vi "WILT.vi"() -> ()   [LabVIEW 2016] (continued)
        n1786 = call "WILT Station Controller.vi"("Station Number"=w3862, "GUI Aisle in"=w3864, "Drying Time (Min)"=w3846, "Current Threshold"=w3852, "Station Test State In"=w3857, "Error In"=w3861, "Aisle Location Index"=w3859, "Cool Down Period (seconds)"=w3847, "Disable Flood Check"=w3842, "Delay After Cutout (sec)"=w3844, "Previous Run Statistics"=w3848, "Send Restart Every? (Sec)"=w3849, "Agilent Valve and Switch Locations"=w3853, "Injection Times"=w3855, "Enable Start Retry"=w3850, "Day/Night Cycle"=w3854, "Final Start Presses"=w3843, "Semaphore"=w3845) -> ("GUI Aisle 1"=w3863:T3[], "Test Station Out"=w3858:T7, "Enable Start Retry Out"=w3851:bool[], "Error Out"=w3860:errorcluster)  [unwired: 5 in, 1 out]
        n1787 = Bundle By Name(cluster=w3866, "GUI Aisle 3."=w3863, "Station Test State Cluster"=w3858, "Enable Start Retry Array"=w3851) -> (w3865:T24)
        n1788 = call <vilib>:"Add State(s) to Queue__jki_lib_state_machine.vi"("State(s) in (\"\")"=w3868) -> ("States Out"=w3867:string)  [unwired: 14 in]
      }
      frame "Station 42" {
        w3886 = 9  # Aisle Location Index
        w3889 = u32 42  # Station Number
        # "Control the state of station 42"
        n1789 = Unbundle By Name(w3893) -> ("Enable Start Retry Array"=w3878:bool[], "Agilent Switches"=w3880:T2[], "GUI Aisle 3."=w3891:T3[], "Drying Time (Min)"=w3873:dbl[], "Current Threshold"=w3879:dbl, "Station Test State Cluster"=w3884:T7, "Station Timeout Values (1-56) Seconds"=w3874:dbl[], "Send Restart Every? (Sec)"=w3876:dbl, "Injection Times Input"=w3882:T15, "Day/Night Cycle Input"=w3881:T11)
        n1790 = local read "Delay After Cutout (Sec)"() -> (w3871:dbl)
        n1791 = local read "Previous Run Statistics"() -> (w3875:T9[])
        n1792 = local read "Agilent Semaphore"() -> (w3872:T1[])
        n1793 = local read "Disable Flood Check"() -> (w3869:bool)
        n1794 = local read "Final Start Presses"() -> (w3870:i32)
        n1795 = call "WILT Station Controller.vi"("Station Number"=w3889, "GUI Aisle in"=w3891, "Drying Time (Min)"=w3873, "Current Threshold"=w3879, "Station Test State In"=w3884, "Error In"=w3888, "Aisle Location Index"=w3886, "Cool Down Period (seconds)"=w3874, "Disable Flood Check"=w3869, "Delay After Cutout (sec)"=w3871, "Previous Run Statistics"=w3875, "Send Restart Every? (Sec)"=w3876, "Agilent Valve and Switch Locations"=w3880, "Injection Times"=w3882, "Enable Start Retry"=w3878, "Day/Night Cycle"=w3881, "Final Start Presses"=w3870, "Semaphore"=w3872) -> ("GUI Aisle 1"=w3890:T3[], "Test Station Out"=w3885:T7, "Enable Start Retry Out"=w3877:bool[], "Error Out"=w3887:errorcluster)  [unwired: 5 in, 1 out]
        n1796 = Bundle By Name(cluster=w3893, "GUI Aisle 3."=w3890, "Station Test State Cluster"=w3885, "Enable Start Retry Array"=w3877) -> (w3892:T24)
        n1797 = call <vilib>:"Add State(s) to Queue__jki_lib_state_machine.vi"("State(s) in (\"\")"=w3895) -> ("States Out"=w3894:string)  [unwired: 14 in]
      }
      frame "Station 43" {
        w3913 = 10  # Aisle Location Index
        w3916 = u32 43  # Station Number
        # "Control the state of station 43"
        n1798 = Unbundle By Name(w3920) -> ("Enable Start Retry Array"=w3905:bool[], "Agilent Switches"=w3907:T2[], "GUI Aisle 3."=w3918:T3[], "Drying Time (Min)"=w3900:dbl[], "Current Threshold"=w3906:dbl, "Station Test State Cluster"=w3911:T7, "Station Timeout Values (1-56) Seconds"=w3901:dbl[], "Send Restart Every? (Sec)"=w3903:dbl, "Injection Times Input"=w3909:T15, "Day/Night Cycle Input"=w3908:T11)
        n1799 = local read "Previous Run Statistics"() -> (w3902:T9[])
        n1800 = local read "Delay After Cutout (Sec)"() -> (w3898:dbl)
        n1801 = local read "Disable Flood Check"() -> (w3896:bool)
        n1802 = local read "Agilent Semaphore"() -> (w3899:T1[])
        n1803 = local read "Final Start Presses"() -> (w3897:i32)
        n1804 = call "WILT Station Controller.vi"("Station Number"=w3916, "GUI Aisle in"=w3918, "Drying Time (Min)"=w3900, "Current Threshold"=w3906, "Station Test State In"=w3911, "Error In"=w3915, "Aisle Location Index"=w3913, "Cool Down Period (seconds)"=w3901, "Disable Flood Check"=w3896, "Delay After Cutout (sec)"=w3898, "Previous Run Statistics"=w3902, "Send Restart Every? (Sec)"=w3903, "Agilent Valve and Switch Locations"=w3907, "Injection Times"=w3909, "Enable Start Retry"=w3905, "Day/Night Cycle"=w3908, "Final Start Presses"=w3897, "Semaphore"=w3899) -> ("GUI Aisle 1"=w3917:T3[], "Test Station Out"=w3912:T7, "Enable Start Retry Out"=w3904:bool[], "Error Out"=w3914:errorcluster)  [unwired: 5 in, 1 out]
        n1805 = call <vilib>:"Add State(s) to Queue__jki_lib_state_machine.vi"("State(s) in (\"\")"=w3922) -> ("States Out"=w3921:string)  [unwired: 14 in]
        n1806 = Bundle By Name(cluster=w3920, "GUI Aisle 3."=w3917, "Station Test State Cluster"=w3912, "Enable Start Retry Array"=w3904) -> (w3919:T24)
      }
      frame "Station 44" {
        w3940 = 11  # Aisle Location Index
        w3943 = u32 44  # Station Number
        # "Control the state of station 44"
        n1807 = Unbundle By Name(w3947) -> ("Enable Start Retry Array"=w3932:bool[], "Agilent Switches"=w3934:T2[], "GUI Aisle 3."=w3945:T3[], "Drying Time (Min)"=w3927:dbl[], "Current Threshold"=w3933:dbl, "Station Test State Cluster"=w3938:T7, "Station Timeout Values (1-56) Seconds"=w3928:dbl[], "Send Restart Every? (Sec)"=w3930:dbl, "Injection Times Input"=w3936:T15, "Day/Night Cycle Input"=w3935:T11)
        n1808 = local read "Previous Run Statistics"() -> (w3929:T9[])
        n1809 = local read "Disable Flood Check"() -> (w3923:bool)
        n1810 = local read "Delay After Cutout (Sec)"() -> (w3925:dbl)
        n1811 = local read "Agilent Semaphore"() -> (w3926:T1[])
        n1812 = local read "Final Start Presses"() -> (w3924:i32)
        n1813 = call "WILT Station Controller.vi"("Station Number"=w3943, "GUI Aisle in"=w3945, "Drying Time (Min)"=w3927, "Current Threshold"=w3933, "Station Test State In"=w3938, "Error In"=w3942, "Aisle Location Index"=w3940, "Cool Down Period (seconds)"=w3928, "Disable Flood Check"=w3923, "Delay After Cutout (sec)"=w3925, "Previous Run Statistics"=w3929, "Send Restart Every? (Sec)"=w3930, "Agilent Valve and Switch Locations"=w3934, "Injection Times"=w3936, "Enable Start Retry"=w3932, "Day/Night Cycle"=w3935, "Final Start Presses"=w3924, "Semaphore"=w3926) -> ("GUI Aisle 1"=w3944:T3[], "Test Station Out"=w3939:T7, "Enable Start Retry Out"=w3931:bool[], "Error Out"=w3941:errorcluster)  [unwired: 5 in, 1 out]
        n1814 = Bundle By Name(cluster=w3947, "GUI Aisle 3."=w3944, "Station Test State Cluster"=w3939, "Enable Start Retry Array"=w3931) -> (w3946:T24)
        n1815 = call <vilib>:"Add State(s) to Queue__jki_lib_state_machine.vi"("State(s) in (\"\")"=w3949) -> ("States Out"=w3948:string)  [unwired: 14 in]
      }
      frame "Station 45" {
        w3967 = 0  # Aisle Location Index
        w3970 = u32 45  # Station Number
        # "Control the state of station 45"
        n1816 = Unbundle By Name(w3974) -> ("Enable Start Retry Array"=w3958:bool[], "Agilent Switches"=w3961:T2[], "GUI Aisle 4."=w3972:T3[], "Drying Time (Min)"=w3954:dbl[], "Current Threshold"=w3960:dbl, "Station Test State Cluster"=w3965:T7, "Station Timeout Values (1-56) Seconds"=w3955:dbl[], "Send Restart Every? (Sec)"=w3957:dbl, "Injection Times Input"=w3963:T15, "Day/Night Cycle Input"=w3962:T11)
        n1817 = local read "Delay After Cutout (Sec)"() -> (w3952:dbl)
        n1818 = local read "Previous Run Statistics"() -> (w3956:T9[])
        n1819 = local read "Agilent Semaphore"() -> (w3953:T1[])
        n1820 = local read "Disable Flood Check"() -> (w3950:bool)
        n1821 = local read "Final Start Presses"() -> (w3951:i32)
        n1822 = call "WILT Station Controller.vi"("Station Number"=w3970, "GUI Aisle in"=w3972, "Drying Time (Min)"=w3954, "Current Threshold"=w3960, "Station Test State In"=w3965, "Error In"=w3969, "Aisle Location Index"=w3967, "Cool Down Period (seconds)"=w3955, "Disable Flood Check"=w3950, "Delay After Cutout (sec)"=w3952, "Previous Run Statistics"=w3956, "Send Restart Every? (Sec)"=w3957, "Agilent Valve and Switch Locations"=w3961, "Injection Times"=w3963, "Enable Start Retry"=w3958, "Day/Night Cycle"=w3962, "Final Start Presses"=w3951, "Semaphore"=w3953) -> ("GUI Aisle 1"=w3971:T3[], "Test Station Out"=w3966:T7, "Enable Start Retry Out"=w3959:bool[], "Error Out"=w3968:errorcluster)  [unwired: 5 in, 1 out]
        n1823 = Bundle By Name(cluster=w3974, "GUI Aisle 4."=w3971, "Station Test State Cluster"=w3966, "Enable Start Retry Array"=w3959) -> (w3973:T24)
        n1824 = call <vilib>:"Add State(s) to Queue__jki_lib_state_machine.vi"("State(s) in (\"\")"=w3976) -> ("States Out"=w3975:string)  [unwired: 14 in]
      }
      frame "Station 46" {
        w3994 = 1  # Aisle Location Index
        w3997 = u32 46  # Station Number
        # "Control the state of station 46"
        n1825 = Unbundle By Name(w4001) -> ("Enable Start Retry Array"=w3985:bool[], "Agilent Switches"=w3988:T2[], "GUI Aisle 4."=w3999:T3[], "Drying Time (Min)"=w3981:dbl[], "Current Threshold"=w3987:dbl, "Station Test State Cluster"=w3992:T7, "Station Timeout Values (1-56) Seconds"=w3982:dbl[], "Send Restart Every? (Sec)"=w3984:dbl, "Injection Times Input"=w3990:T15, "Day/Night Cycle Input"=w3989:T11)
        n1826 = local read "Delay After Cutout (Sec)"() -> (w3979:dbl)
        n1827 = local read "Final Start Presses"() -> (w3978:i32)
        n1828 = local read "Agilent Semaphore"() -> (w3980:T1[])
        n1829 = local read "Previous Run Statistics"() -> (w3983:T9[])
        n1830 = local read "Disable Flood Check"() -> (w3977:bool)
        n1831 = call "WILT Station Controller.vi"("Station Number"=w3997, "GUI Aisle in"=w3999, "Drying Time (Min)"=w3981, "Current Threshold"=w3987, "Station Test State In"=w3992, "Error In"=w3996, "Aisle Location Index"=w3994, "Cool Down Period (seconds)"=w3982, "Disable Flood Check"=w3977, "Delay After Cutout (sec)"=w3979, "Previous Run Statistics"=w3983, "Send Restart Every? (Sec)"=w3984, "Agilent Valve and Switch Locations"=w3988, "Injection Times"=w3990, "Enable Start Retry"=w3985, "Day/Night Cycle"=w3989, "Final Start Presses"=w3978, "Semaphore"=w3980) -> ("GUI Aisle 1"=w3998:T3[], "Test Station Out"=w3993:T7, "Enable Start Retry Out"=w3986:bool[], "Error Out"=w3995:errorcluster)  [unwired: 5 in, 1 out]
        n1832 = Bundle By Name(cluster=w4001, "GUI Aisle 4."=w3998, "Station Test State Cluster"=w3993, "Enable Start Retry Array"=w3986) -> (w4000:T24)
        n1833 = call <vilib>:"Add State(s) to Queue__jki_lib_state_machine.vi"("State(s) in (\"\")"=w4003) -> ("States Out"=w4002:string)  [unwired: 14 in]
      }
      frame "Station 47" {
        w4021 = 2  # Aisle Location Index
        w4024 = u32 47  # Station Number
        # "Control the state of station 47"
        n1834 = Unbundle By Name(w4028) -> ("Enable Start Retry Array"=w4012:bool[], "Agilent Switches"=w4016:T2[], "GUI Aisle 4."=w4026:T3[], "Drying Time (Min)"=w4009:dbl[], "Current Threshold"=w4015:dbl, "Station Test State Cluster"=w4019:T7, "Station Timeout Values (1-56) Seconds"=w4008:dbl[], "Send Restart Every? (Sec)"=w4011:dbl, "Injection Times Input"=w4017:T15, "Day/Night Cycle Input"=w4014:T11)
        n1835 = local read "Delay After Cutout (Sec)"() -> (w4006:dbl)
        n1836 = local read "Final Start Presses"() -> (w4005:i32)
        n1837 = local read "Agilent Semaphore"() -> (w4007:T1[])
        n1838 = local read "Previous Run Statistics"() -> (w4010:T9[])
        n1839 = local read "Disable Flood Check"() -> (w4004:bool)
        n1840 = call "WILT Station Controller.vi"("Station Number"=w4024, "GUI Aisle in"=w4026, "Drying Time (Min)"=w4009, "Current Threshold"=w4015, "Station Test State In"=w4019, "Error In"=w4023, "Aisle Location Index"=w4021, "Cool Down Period (seconds)"=w4008, "Disable Flood Check"=w4004, "Delay After Cutout (sec)"=w4006, "Previous Run Statistics"=w4010, "Send Restart Every? (Sec)"=w4011, "Agilent Valve and Switch Locations"=w4016, "Injection Times"=w4017, "Enable Start Retry"=w4012, "Day/Night Cycle"=w4014, "Final Start Presses"=w4005, "Semaphore"=w4007) -> ("GUI Aisle 1"=w4025:T3[], "Test Station Out"=w4020:T7, "Enable Start Retry Out"=w4013:bool[], "Error Out"=w4022:errorcluster)  [unwired: 5 in, 1 out]
        n1841 = Bundle By Name(cluster=w4028, "GUI Aisle 4."=w4025, "Station Test State Cluster"=w4020, "Enable Start Retry Array"=w4013) -> (w4027:T24)
        n1842 = call <vilib>:"Add State(s) to Queue__jki_lib_state_machine.vi"("State(s) in (\"\")"=w4030) -> ("States Out"=w4029:string)  [unwired: 14 in]
      }
      frame "Station 48" {
        w4048 = 3  # Aisle Location Index
        w4051 = u32 48  # Station Number
        # "Control the state of station 48"
        n1843 = Unbundle By Name(w4055) -> ("Enable Start Retry Array"=w4040:bool[], "Agilent Switches"=w4042:T2[], "GUI Aisle 4."=w4053:T3[], "Drying Time (Min)"=w4035:dbl[], "Current Threshold"=w4041:dbl, "Station Test State Cluster"=w4046:T7, "Station Timeout Values (1-56) Seconds"=w4036:dbl[], "Send Restart Every? (Sec)"=w4038:dbl, "Injection Times Input"=w4044:T15, "Day/Night Cycle Input"=w4043:T11)
        n1844 = local read "Previous Run Statistics"() -> (w4037:T9[])
        n1845 = local read "Disable Flood Check"() -> (w4031:bool)
        n1846 = local read "Delay After Cutout (Sec)"() -> (w4033:dbl)
        n1847 = local read "Agilent Semaphore"() -> (w4034:T1[])
        n1848 = local read "Final Start Presses"() -> (w4032:i32)
        n1849 = call "WILT Station Controller.vi"("Station Number"=w4051, "GUI Aisle in"=w4053, "Drying Time (Min)"=w4035, "Current Threshold"=w4041, "Station Test State In"=w4046, "Error In"=w4050, "Aisle Location Index"=w4048, "Cool Down Period (seconds)"=w4036, "Disable Flood Check"=w4031, "Delay After Cutout (sec)"=w4033, "Previous Run Statistics"=w4037, "Send Restart Every? (Sec)"=w4038, "Agilent Valve and Switch Locations"=w4042, "Injection Times"=w4044, "Enable Start Retry"=w4040, "Day/Night Cycle"=w4043, "Final Start Presses"=w4032, "Semaphore"=w4034) -> ("GUI Aisle 1"=w4052:T3[], "Test Station Out"=w4047:T7, "Enable Start Retry Out"=w4039:bool[], "Error Out"=w4049:errorcluster)  [unwired: 5 in, 1 out]
        n1850 = Bundle By Name(cluster=w4055, "GUI Aisle 4."=w4052, "Station Test State Cluster"=w4047, "Enable Start Retry Array"=w4039) -> (w4054:T24)
        n1851 = call <vilib>:"Add State(s) to Queue__jki_lib_state_machine.vi"("State(s) in (\"\")"=w4057) -> ("States Out"=w4056:string)  [unwired: 14 in]
      }
      frame "Station 49" {
        w4075 = 4  # Aisle Location Index
        w4078 = u32 49  # Station Number
        # "Control the state of station 49"
        n1852 = Unbundle By Name(w4082) -> ("Enable Start Retry Array"=w4067:bool[], "Agilent Switches"=w4069:T2[], "GUI Aisle 4."=w4080:T3[], "Drying Time (Min)"=w4062:dbl[], "Current Threshold"=w4068:dbl, "Station Test State Cluster"=w4073:T7, "Station Timeout Values (1-56) Seconds"=w4063:dbl[], "Send Restart Every? (Sec)"=w4065:dbl, "Injection Times Input"=w4071:T15, "Day/Night Cycle Input"=w4070:T11)
        n1853 = local read "Previous Run Statistics"() -> (w4064:T9[])
        n1854 = local read "Disable Flood Check"() -> (w4058:bool)
        n1855 = local read "Delay After Cutout (Sec)"() -> (w4060:dbl)
        n1856 = local read "Final Start Presses"() -> (w4059:i32)
        n1857 = local read "Agilent Semaphore"() -> (w4061:T1[])
        n1858 = call "WILT Station Controller.vi"("Station Number"=w4078, "GUI Aisle in"=w4080, "Drying Time (Min)"=w4062, "Current Threshold"=w4068, "Station Test State In"=w4073, "Error In"=w4077, "Aisle Location Index"=w4075, "Cool Down Period (seconds)"=w4063, "Disable Flood Check"=w4058, "Delay After Cutout (sec)"=w4060, "Previous Run Statistics"=w4064, "Send Restart Every? (Sec)"=w4065, "Agilent Valve and Switch Locations"=w4069, "Injection Times"=w4071, "Enable Start Retry"=w4067, "Day/Night Cycle"=w4070, "Final Start Presses"=w4059, "Semaphore"=w4061) -> ("GUI Aisle 1"=w4079:T3[], "Test Station Out"=w4074:T7, "Enable Start Retry Out"=w4066:bool[], "Error Out"=w4076:errorcluster)  [unwired: 5 in, 1 out]
        n1859 = Bundle By Name(cluster=w4082, "GUI Aisle 4."=w4079, "Station Test State Cluster"=w4074, "Enable Start Retry Array"=w4066) -> (w4081:T24)
        n1860 = call <vilib>:"Add State(s) to Queue__jki_lib_state_machine.vi"("State(s) in (\"\")"=w4084) -> ("States Out"=w4083:string)  [unwired: 14 in]
      }
      frame "Station 50" {
        w4102 = 5  # Aisle Location Index
        w4105 = u32 50  # Station Number
        # "Control the state of station 50"
        n1861 = Unbundle By Name(w4109) -> ("Enable Start Retry Array"=w4094:bool[], "Agilent Switches"=w4096:T2[], "GUI Aisle 4."=w4107:T3[], "Drying Time (Min)"=w4089:dbl[], "Current Threshold"=w4095:dbl, "Station Test State Cluster"=w4100:T7, "Station Timeout Values (1-56) Seconds"=w4090:dbl[], "Send Restart Every? (Sec)"=w4092:dbl, "Injection Times Input"=w4098:T15, "Day/Night Cycle Input"=w4097:T11)
        n1862 = local read "Previous Run Statistics"() -> (w4091:T9[])
        n1863 = local read "Disable Flood Check"() -> (w4085:bool)
        n1864 = local read "Delay After Cutout (Sec)"() -> (w4087:dbl)
        n1865 = local read "Final Start Presses"() -> (w4086:i32)
        n1866 = local read "Agilent Semaphore"() -> (w4088:T1[])
        n1867 = call "WILT Station Controller.vi"("Station Number"=w4105, "GUI Aisle in"=w4107, "Drying Time (Min)"=w4089, "Current Threshold"=w4095, "Station Test State In"=w4100, "Error In"=w4104, "Aisle Location Index"=w4102, "Cool Down Period (seconds)"=w4090, "Disable Flood Check"=w4085, "Delay After Cutout (sec)"=w4087, "Previous Run Statistics"=w4091, "Send Restart Every? (Sec)"=w4092, "Agilent Valve and Switch Locations"=w4096, "Injection Times"=w4098, "Enable Start Retry"=w4094, "Day/Night Cycle"=w4097, "Final Start Presses"=w4086, "Semaphore"=w4088) -> ("GUI Aisle 1"=w4106:T3[], "Test Station Out"=w4101:T7, "Enable Start Retry Out"=w4093:bool[], "Error Out"=w4103:errorcluster)  [unwired: 5 in, 1 out]
        n1868 = Bundle By Name(cluster=w4109, "GUI Aisle 4."=w4106, "Station Test State Cluster"=w4101, "Enable Start Retry Array"=w4093) -> (w4108:T24)
        n1869 = call <vilib>:"Add State(s) to Queue__jki_lib_state_machine.vi"("State(s) in (\"\")"=w4111) -> ("States Out"=w4110:string)  [unwired: 14 in]
      }
      frame "Station 51" {
        w4129 = 6  # Aisle Location Index
        w4132 = u32 51  # Station Number
        # "Control the state of station 51"
        n1870 = Unbundle By Name(w4136) -> ("Enable Start Retry Array"=w4121:bool[], "Agilent Switches"=w4123:T2[], "GUI Aisle 4."=w4134:T3[], "Drying Time (Min)"=w4116:dbl[], "Current Threshold"=w4122:dbl, "Station Test State Cluster"=w4127:T7, "Station Timeout Values (1-56) Seconds"=w4117:dbl[], "Send Restart Every? (Sec)"=w4119:dbl, "Injection Times Input"=w4125:T15, "Day/Night Cycle Input"=w4124:T11)
        n1871 = local read "Delay After Cutout (Sec)"() -> (w4114:dbl)
        n1872 = local read "Final Start Presses"() -> (w4113:i32)
        n1873 = local read "Agilent Semaphore"() -> (w4115:T1[])
        n1874 = local read "Previous Run Statistics"() -> (w4118:T9[])
        n1875 = local read "Disable Flood Check"() -> (w4112:bool)
        n1876 = call "WILT Station Controller.vi"("Station Number"=w4132, "GUI Aisle in"=w4134, "Drying Time (Min)"=w4116, "Current Threshold"=w4122, "Station Test State In"=w4127, "Error In"=w4131, "Aisle Location Index"=w4129, "Cool Down Period (seconds)"=w4117, "Disable Flood Check"=w4112, "Delay After Cutout (sec)"=w4114, "Previous Run Statistics"=w4118, "Send Restart Every? (Sec)"=w4119, "Agilent Valve and Switch Locations"=w4123, "Injection Times"=w4125, "Enable Start Retry"=w4121, "Day/Night Cycle"=w4124, "Final Start Presses"=w4113, "Semaphore"=w4115) -> ("GUI Aisle 1"=w4133:T3[], "Test Station Out"=w4128:T7, "Enable Start Retry Out"=w4120:bool[], "Error Out"=w4130:errorcluster)  [unwired: 5 in, 1 out]
        n1877 = Bundle By Name(cluster=w4136, "GUI Aisle 4."=w4133, "Station Test State Cluster"=w4128, "Enable Start Retry Array"=w4120) -> (w4135:T24)
        n1878 = call <vilib>:"Add State(s) to Queue__jki_lib_state_machine.vi"("State(s) in (\"\")"=w4138) -> ("States Out"=w4137:string)  [unwired: 14 in]
      }
      frame "Station 52" {
        w4156 = 7  # Aisle Location Index
        w4159 = u32 52  # Station Number
        # "Control the state of station 52"
        n1879 = Unbundle By Name(w4163) -> ("Enable Start Retry Array"=w4148:bool[], "Agilent Switches"=w4150:T2[], "GUI Aisle 4."=w4161:T3[], "Drying Time (Min)"=w4143:dbl[], "Current Threshold"=w4149:dbl, "Station Test State Cluster"=w4154:T7, "Station Timeout Values (1-56) Seconds"=w4144:dbl[], "Send Restart Every? (Sec)"=w4146:dbl, "Injection Times Input"=w4152:T15, "Day/Night Cycle Input"=w4151:T11)
        n1880 = local read "Previous Run Statistics"() -> (w4145:T9[])
        n1881 = local read "Disable Flood Check"() -> (w4139:bool)
        n1882 = local read "Delay After Cutout (Sec)"() -> (w4141:dbl)
        n1883 = local read "Final Start Presses"() -> (w4140:i32)
        n1884 = local read "Agilent Semaphore"() -> (w4142:T1[])
        n1885 = call "WILT Station Controller.vi"("Station Number"=w4159, "GUI Aisle in"=w4161, "Drying Time (Min)"=w4143, "Current Threshold"=w4149, "Station Test State In"=w4154, "Error In"=w4158, "Aisle Location Index"=w4156, "Cool Down Period (seconds)"=w4144, "Disable Flood Check"=w4139, "Delay After Cutout (sec)"=w4141, "Previous Run Statistics"=w4145, "Send Restart Every? (Sec)"=w4146, "Agilent Valve and Switch Locations"=w4150, "Injection Times"=w4152, "Enable Start Retry"=w4148, "Day/Night Cycle"=w4151, "Final Start Presses"=w4140, "Semaphore"=w4142) -> ("GUI Aisle 1"=w4160:T3[], "Test Station Out"=w4155:T7, "Enable Start Retry Out"=w4147:bool[], "Error Out"=w4157:errorcluster)  [unwired: 5 in, 1 out]
        n1886 = Bundle By Name(cluster=w4163, "GUI Aisle 4."=w4160, "Station Test State Cluster"=w4155, "Enable Start Retry Array"=w4147) -> (w4162:T24)
        n1887 = call <vilib>:"Add State(s) to Queue__jki_lib_state_machine.vi"("State(s) in (\"\")"=w4165) -> ("States Out"=w4164:string)  [unwired: 14 in]
      }
      frame "Station 53" {
        w4183 = 8  # Aisle Location Index
        w4186 = u32 53  # Station Number
        # "Control the state of station 53"
        n1888 = Unbundle By Name(w4190) -> ("Enable Start Retry Array"=w4175:bool[], "Agilent Switches"=w4177:T2[], "GUI Aisle 4."=w4188:T3[], "Drying Time (Min)"=w4170:dbl[], "Current Threshold"=w4176:dbl, "Station Test State Cluster"=w4181:T7, "Station Timeout Values (1-56) Seconds"=w4171:dbl[], "Send Restart Every? (Sec)"=w4173:dbl, "Injection Times Input"=w4179:T15, "Day/Night Cycle Input"=w4178:T11)
        n1889 = local read "Previous Run Statistics"() -> (w4172:T9[])
        n1890 = local read "Delay After Cutout (Sec)"() -> (w4168:dbl)
        n1891 = local read "Final Start Presses"() -> (w4167:i32)
        n1892 = local read "Agilent Semaphore"() -> (w4169:T1[])
        n1893 = local read "Disable Flood Check"() -> (w4166:bool)
        n1894 = call "WILT Station Controller.vi"("Station Number"=w4186, "GUI Aisle in"=w4188, "Drying Time (Min)"=w4170, "Current Threshold"=w4176, "Station Test State In"=w4181, "Error In"=w4185, "Aisle Location Index"=w4183, "Cool Down Period (seconds)"=w4171, "Disable Flood Check"=w4166, "Delay After Cutout (sec)"=w4168, "Previous Run Statistics"=w4172, "Send Restart Every? (Sec)"=w4173, "Agilent Valve and Switch Locations"=w4177, "Injection Times"=w4179, "Enable Start Retry"=w4175, "Day/Night Cycle"=w4178, "Final Start Presses"=w4167, "Semaphore"=w4169) -> ("GUI Aisle 1"=w4187:T3[], "Test Station Out"=w4182:T7, "Enable Start Retry Out"=w4174:bool[], "Error Out"=w4184:errorcluster)  [unwired: 5 in, 1 out]
        n1895 = Bundle By Name(cluster=w4190, "GUI Aisle 4."=w4187, "Station Test State Cluster"=w4182, "Enable Start Retry Array"=w4174) -> (w4189:T24)
        n1896 = call <vilib>:"Add State(s) to Queue__jki_lib_state_machine.vi"("State(s) in (\"\")"=w4192) -> ("States Out"=w4191:string)  [unwired: 14 in]
      }
      frame "Station 54" {
        w4210 = 9  # Aisle Location Index
        w4213 = u32 54  # Station Number
        # "Control the state of station 54"
        n1897 = Unbundle By Name(w4217) -> ("Enable Start Retry Array"=w4201:bool[], "Agilent Switches"=w4204:T2[], "GUI Aisle 4."=w4215:T3[], "Drying Time (Min)"=w4197:dbl[], "Current Threshold"=w4203:dbl, "Station Test State Cluster"=w4208:T7, "Station Timeout Values (1-56) Seconds"=w4198:dbl[], "Send Restart Every? (Sec)"=w4200:dbl, "Injection Times Input"=w4206:T15, "Day/Night Cycle Input"=w4205:T11)
        n1898 = local read "Delay After Cutout (Sec)"() -> (w4195:dbl)
        n1899 = local read "Previous Run Statistics"() -> (w4199:T9[])
        n1900 = local read "Disable Flood Check"() -> (w4193:bool)
        n1901 = local read "Agilent Semaphore"() -> (w4196:T1[])
        n1902 = local read "Final Start Presses"() -> (w4194:i32)
        n1903 = call "WILT Station Controller.vi"("Station Number"=w4213, "GUI Aisle in"=w4215, "Drying Time (Min)"=w4197, "Current Threshold"=w4203, "Station Test State In"=w4208, "Error In"=w4212, "Aisle Location Index"=w4210, "Cool Down Period (seconds)"=w4198, "Disable Flood Check"=w4193, "Delay After Cutout (sec)"=w4195, "Previous Run Statistics"=w4199, "Send Restart Every? (Sec)"=w4200, "Agilent Valve and Switch Locations"=w4204, "Injection Times"=w4206, "Enable Start Retry"=w4201, "Day/Night Cycle"=w4205, "Final Start Presses"=w4194, "Semaphore"=w4196) -> ("GUI Aisle 1"=w4214:T3[], "Test Station Out"=w4209:T7, "Enable Start Retry Out"=w4202:bool[], "Error Out"=w4211:errorcluster)  [unwired: 5 in, 1 out]
        n1904 = Bundle By Name(cluster=w4217, "GUI Aisle 4."=w4214, "Station Test State Cluster"=w4209, "Enable Start Retry Array"=w4202) -> (w4216:T24)
        n1905 = call <vilib>:"Add State(s) to Queue__jki_lib_state_machine.vi"("State(s) in (\"\")"=w4219) -> ("States Out"=w4218:string)  [unwired: 14 in]
      }
      frame "Station 55" {
        w4237 = 10  # Aisle Location Index
        w4240 = u32 55  # Station Number
        # "Control the state of station 55"
        n1906 = Unbundle By Name(w4244) -> ("Enable Start Retry Array"=w4228:bool[], "Agilent Switches"=w4231:T2[], "GUI Aisle 4."=w4242:T3[], "Drying Time (Min)"=w4224:dbl[], "Current Threshold"=w4230:dbl, "Station Test State Cluster"=w4235:T7, "Station Timeout Values (1-56) Seconds"=w4225:dbl[], "Send Restart Every? (Sec)"=w4227:dbl, "Injection Times Input"=w4233:T15, "Day/Night Cycle Input"=w4232:T11)
        n1907 = local read "Delay After Cutout (Sec)"() -> (w4222:dbl)
        n1908 = local read "Agilent Semaphore"() -> (w4223:T1[])
        n1909 = local read "Final Start Presses"() -> (w4221:i32)
        n1910 = local read "Previous Run Statistics"() -> (w4226:T9[])
        n1911 = local read "Disable Flood Check"() -> (w4220:bool)
        n1912 = call "WILT Station Controller.vi"("Station Number"=w4240, "GUI Aisle in"=w4242, "Drying Time (Min)"=w4224, "Current Threshold"=w4230, "Station Test State In"=w4235, "Error In"=w4239, "Aisle Location Index"=w4237, "Cool Down Period (seconds)"=w4225, "Disable Flood Check"=w4220, "Delay After Cutout (sec)"=w4222, "Previous Run Statistics"=w4226, "Send Restart Every? (Sec)"=w4227, "Agilent Valve and Switch Locations"=w4231, "Injection Times"=w4233, "Enable Start Retry"=w4228, "Day/Night Cycle"=w4232, "Final Start Presses"=w4221, "Semaphore"=w4223) -> ("GUI Aisle 1"=w4241:T3[], "Test Station Out"=w4236:T7, "Enable Start Retry Out"=w4229:bool[], "Error Out"=w4238:errorcluster)  [unwired: 5 in, 1 out]
        n1913 = Bundle By Name(cluster=w4244, "GUI Aisle 4."=w4241, "Station Test State Cluster"=w4236, "Enable Start Retry Array"=w4229) -> (w4243:T24)
        n1914 = call <vilib>:"Add State(s) to Queue__jki_lib_state_machine.vi"("State(s) in (\"\")"=w4246) -> ("States Out"=w4245:string)  [unwired: 14 in]
      }
      frame "Station 56" {
        w4264 = 11  # Aisle Location Index
        w4267 = u32 56  # Station Number
        # "Control the state of station 56"
        n1915 = Unbundle By Name(w4271) -> ("Enable Start Retry Array"=w4255:bool[], "Agilent Switches"=w4258:T2[], "GUI Aisle 4."=w4269:T3[], "Drying Time (Min)"=w4251:dbl[], "Current Threshold"=w4257:dbl, "Station Test State Cluster"=w4262:T7, "Station Timeout Values (1-56) Seconds"=w4252:dbl[], "Send Restart Every? (Sec)"=w4254:dbl, "Injection Times Input"=w4260:T15, "Day/Night Cycle Input"=w4259:T11)
        n1916 = local read "Delay After Cutout (Sec)"() -> (w4249:dbl)
        n1917 = local read "Final Start Presses"() -> (w4248:i32)
        n1918 = local read "Agilent Semaphore"() -> (w4250:T1[])
        n1919 = local read "Previous Run Statistics"() -> (w4253:T9[])
        n1920 = local read "Disable Flood Check"() -> (w4247:bool)
        n1921 = call "WILT Station Controller.vi"("Station Number"=w4267, "GUI Aisle in"=w4269, "Drying Time (Min)"=w4251, "Current Threshold"=w4257, "Station Test State In"=w4262, "Error In"=w4266, "Aisle Location Index"=w4264, "Cool Down Period (seconds)"=w4252, "Disable Flood Check"=w4247, "Delay After Cutout (sec)"=w4249, "Previous Run Statistics"=w4253, "Send Restart Every? (Sec)"=w4254, "Agilent Valve and Switch Locations"=w4258, "Injection Times"=w4260, "Enable Start Retry"=w4255, "Day/Night Cycle"=w4259, "Final Start Presses"=w4248, "Semaphore"=w4250) -> ("GUI Aisle 1"=w4268:T3[], "Test Station Out"=w4263:T7, "Enable Start Retry Out"=w4256:bool[], "Error Out"=w4265:errorcluster)  [unwired: 5 in, 1 out]
        n1922 = Bundle By Name(cluster=w4271, "GUI Aisle 4."=w4268, "Station Test State Cluster"=w4263, "Enable Start Retry Array"=w4256) -> (w4270:T24)
        n1923 = call <vilib>:"Add State(s) to Queue__jki_lib_state_machine.vi"("State(s) in (\"\")"=w4273) -> ("States Out"=w4272:string)  [unwired: 14 in]
      }
      frame "Get Agilent Data" {
        n1924 = Unbundle By Name(w4291) -> ("Agilent Switches"=→"Agilent Switches Locations":T2[], "Enable Start Retry Array"=→"Enable Start Retry Array":bool[], "GUI Aisle 4."=w4290:T3[], "GUI Aisle 3."=w4289:T3[], "GUI Aisle 2."=w4288:T3[], "GUI Aisle 1 (SLAT)."=w4287:T3[], "GUI Aisle 1A (SLAT)."=w4286:T3[])
        n1925 = local read "Agilent Data Out"() -> (w4278:T6)
        n1926 = call "WILT Agilent Data To Main Display.vi"("GUI Aisle 4"=w4290, "GUI Aisle 3"=w4289, "GUI Aisle 2"=w4288, "GUI Aisle 1 (SLAT)"=w4287, "Error In"=w4279, "GUI Aisle 1A (SLAT)"=w4286, "Data Array"=w4278) -> ("Agilent Failure"=w4275:bool, "GUI Aisle 4 Out"=w4281:T3[], "GUI Aisle 3 Out"=w4282:T3[], "GUI Aisle 2 Out"=w4283:T3[], "GUI Aisle 1 (SLAT) Out"=w4284:T3[], "GUI Aisle 1A (SLAT) Out"=w4285:T3[], "Error Out"=w4292:errorcluster)  [unwired: 2 in]
        n1927 = case shown="True" w4275 {
          tunnel: ["" ("State(s) in Front (\"\")") "Shutdown All Valves" ("State(s) in Front (\"\")")] -> w4274
          frame False {
          }
          frame True {
          }
        }
        n1928 = Bundle By Name(cluster=w4291, "GUI Aisle 4."=w4281, "GUI Aisle 3."=w4282, "GUI Aisle 2."=w4283, "GUI Aisle 1 (SLAT)."=w4284, "GUI Aisle 1A (SLAT)."=w4285) -> (w4293:T24)
        n1929 = call <vilib>:"Add State(s) to Queue__jki_lib_state_machine.vi"("State(s) in Front (\"\")"=w4274, "State(s) in (\"\")"=w4295) -> ("States Out"=w4294:string)  [unwired: 13 in]
      }
      frame "Update States" {
        n1930 = call "UTILITY E-Time.vi"("error in (no error)"=w4316) -> ("error out"=w4315:errorcluster, "Elapsed Time (sec)"=w4310:dbl)  [unwired: 8 in, 1 out]
        "Elapsed Time." <- w4310
        n1931 = Unbundle By Name(w4317) -> ("Send Restart Every? (Sec)"=→"Send Restart Every? (Sec)":dbl, "Station Test State Cluster"=→"Station Test State Cluster 2":T7, "Injection Times Input"=w4301:T15, "GUI Aisle 4."=w4305:T3[], "GUI Aisle 3."=w4306:T3[], "GUI Aisle 2."=w4307:T3[], "GUI Aisle 1A (SLAT)."=w4308:T3[], "GUI Aisle 1 (SLAT)."=w4309:T3[], "File Locations"=w4313:T17[])
        n1932 = Greater?(x=w4310, y=45.0) -> (0:w4311:bool)
        n1933 = case shown="True" w4311 {
          tunnel: w4310 -> [_ w4324]
          tunnel: [FALSE w4321] -> w4299
          frame False {
          }
          frame True {
            n1934 = Quotient & Remainder(x=w4324, y=300.0) -> (x-y*floor(x/y)=w4322:dbl)  [unwired: 1 out]
            n1935 = Round To Nearest(number=w4322) -> (nearest integer value=w4325:dbl)
            n1936 = Equal To 0?(x=w4325) -> (x = 0?=w4321:bool)
          }
        }
        n1937 = case shown="True" w4299 {
          tunnel: w4315 -> [w4326 w4337]
          tunnel: [w4326 w4330] -> w4314
          tunnel: w4313 -> [_ w4327]
          tunnel: w4305 -> [_ w4336]
          tunnel: w4306 -> [_ w4335]
          tunnel: w4307 -> [_ w4334]
          tunnel: w4309 -> [_ w4333]
          tunnel: w4308 -> [_ w4332]
          tunnel: w4301 -> [_ w4328]
          frame False {
          }
          frame True {
            n1938 = call "WILT Stave Status.vi"("GUI Aisle 4"=w4336, "Operation Type"=enum16{"Write", "Read"}."Write", "File Locations"=w4327, "GUI Aisle 3"=w4335, "GUI Aisle 2"=w4334, "GUI Aisle 1 (SLAT)"=w4333, "Error In"=w4337, "GUI Aisle 1A (SLAT)"=w4332) -> ("Error Out"=w4331:errorcluster)  [unwired: 2 in, 5 out]
            n1939 = call "WILT Watering Times.vi"("Watering Times Input"=w4328, "Execution Type"=enum16{"Write", "Read"}."Write", "Error In"=w4331, "File Locations"=w4327) -> ("Error Out"=w4330:errorcluster)  [unwired: 6 in, 1 out]
          }
        }
        n1940 = Build Array (concatenate)(w4309, w4308, w4307, w4306, w4305) -> (w4303:T3[])
        n1941 = Send Notification(notification=w4303, notifier=w4304) -> (notifier out=w4302:refnum<notifier>)  [unwired: 1 in, 1 out]
        n1942 = call <vilib>:"Add State(s) to Queue__jki_lib_state_machine.vi"("State(s) in (\"\")"=w4319) -> ("States Out"=w4318:string)  [unwired: 14 in]
      }
      frame "Update Display" {
        n1943 = Unbundle By Name(w4346) -> ("GUI Aisle 4."=w4344:T3[], "GUI Aisle 3."=w4343:T3[], "GUI Aisle 2."=w4342:T3[], "GUI Aisle 1A (SLAT)."=w4341:T3[], "GUI Aisle 1 (SLAT)."=w4340:T3[])
        n1944 = local write "GUI Aisle 4."(w4344) -> ()
        n1945 = local write "GUI Aisle 3."(w4343) -> ()
        n1946 = local write "GUI Aisle 2."(w4342) -> ()
        n1947 = local write "GUI Aisle 1A (SLAT)."(w4341) -> ()
        n1948 = local write "GUI Aisle 1 (SLAT)."(w4340) -> ()
        n1949 = call <vilib>:"Add State(s) to Queue__jki_lib_state_machine.vi"("State(s) in (\"\")"=w4348) -> ("States Out"=w4347:string)  [unwired: 14 in]
      }
      frame "Update Filenames" {
        # "This is updated from the \nprepare and save loop in the daq sm"
        n1950 = local read "File Locations"() -> (w4350:T17[])
        n1951 = Bundle By Name(cluster=w4353, "File Locations"=w4350) -> (w4354:T24)
        n1952 = call <vilib>:"Add State(s) to Queue__jki_lib_state_machine.vi"("State(s) in (\"\")"=w4352) -> ("States Out"=w4351:string)  [unwired: 14 in]
      }
    }
    "Exit Signal" <- w87
    n1953 = case shown="True" "Debug 2" {
      tunnel: w84 -> [_ w102]
      tunnel: [w97 w99] -> w85
      tunnel: w86 -> [w97 w101]
      frame False {
      }
      frame True {
        n1954 = Build Array (concatenate)(w101, w102) -> (w98:string[])
        "Test State array 2" <- w98
        n1955 = Array Size(array=w98) -> (size(s)=w100:i32)
        n1956 = case shown="100" w100 {
          tunnel: [w103 w106] -> w99
          tunnel: w98 -> [w103 w107]
          frame 0, Default {
          }
          frame 100 {
            n1957 = Delete From Array(array=w107, length=5, index=0) -> (array with subset deleted=w106:string[])  [unwired: 1 out]
          }
        }
      }
    }
  }
  n1958 = register-events(w44) -> (reference out=w43:refnum<event-registration>)  [unwired: 2 in, 1 out]
  n1959 = call <vilib>:"Add State(s) to Queue__jki_lib_state_machine.vi"("State(s) in (\"\")"="Data: Initialize") -> ("States Out"=w48:string)  [unwired: 14 in]
  n1960 = call <vilib>:"Add State(s) to Queue__jki_lib_state_machine.vi"("State(s) in (\"\")"="Data: Initialize") -> ("States Out"=w50:string)  [unwired: 14 in]
  n1961 = call <vilib>:"Add State(s) to Queue__jki_lib_state_machine.vi"("State(s) in (\"\")"="Data: Initialize") -> ("States Out"=w58:string)  [unwired: 14 in]
  n1962 = Merge Errors(w23, w22, w21, w20, w19) -> (w18:errorcluster)
  n1963 = call <vilib>:"Add State(s) to Queue__jki_lib_state_machine.vi"("State(s) in (\"\")"="Data: Initialize") -> ("States Out"=w53:string)  [unwired: 14 in]
  n1964 = while "DAQ State Machine" {
    shift-right: [w4365] -> _
    shift-left: _ -> [w4364]
    shift-right: [w4368] -> _
    shift-left: _ -> [w4363]
    shift-right: [w4367] -> _
    shift-left: w58 -> [w4369]
    shift-right: [w4360] -> _
    shift-left: string[] [] -> [w4361]
    stop <- w4366 stop-if-true
    # "DAQ State Machine"
    n1965 = call <vilib>:"Parse State Queue__jki_lib_state_machine.vi"("State Queue"=w4369, "Error In (no error)"=w4363) -> ("Remaining States"=w4371:string, "Current State"=w4362:string, "Arguments"=w4370:string)  [unwired: 11 in]
    n1966 = Multiply(x=1000, y="Scan Rate (Seconds)") -> (x*y=w4356:i32)
    n1967 = case shown="\"Read Agilents\"" w4362 {
      selector: w4362 -> [_ _ w4410 _ _ _ _ _ _]
      tunnel: w4371 -> [w4389 w4409 w4414 w4426 w4431 w4435 w4442 w4450 w4461]
      tunnel: w4370 -> [_ _ _ _ _ _ _ _ _]
      tunnel: w4364 -> [w4387 w4406 w4412 w4423 w4429 w4432 _ w4447 w4457]
      tunnel: [w4386 w4407 w4416 errorcluster {"status"=FALSE, "code"=0, "source"=""} ("error out") w4428 w4433 w4439 w4448 w4454] -> w4368
      tunnel: w4363 -> [w4385 w4407 w4415 w4422 w4428 w4433 w4439 w4448 w4454]
      tunnel: [w4388 w4408 w4413 w4425 w4430 w4434 w4441 w4449 w4460] -> w4367
      tunnel: [_ _ _ _ TRUE _ _ _ _] -> w4366
      tunnel: [w4384 w4406 w4412 w4423 w4429 w4432 w4440 w4447 w4456] -> w4365
      tunnel: w4356 -> [w4383 _ _ _ _ _ _ _ _]
      frame "", "Idle" {
        n1968 = event shown="[0] Timeout" {
          selector: _ -> [_ _ _]
          dyn-events: _ -> [_ _ _]
          timeout: w4383 -> [_ _ _]
          tunnel: w4389 -> [w4394 w4397 w4405]
          tunnel: [w4393 w4396 w4404] -> w4388
          tunnel: w4387 -> [w4391 w4399 w4402]
          tunnel: [w4392 w4398 w4403] -> w4386
          tunnel: w4385 -> [w4392 w4398 w4403]
          tunnel: [w4391 w4399 w4402] -> w4384
          event Timeout {
            n1969 = event-data() -> ()  [unwired: 1 in, 1 out]
            n1970 = call <vilib>:"Add State(s) to Queue__jki_lib_state_machine.vi"("State(s) in Front (\"\")"="Read Agilents" ("State(s) in Front (\"\")"), "State(s) in (\"\")"=w4394) -> ("States Out"=w4393:string)  [unwired: 13 in]
          }
          event "ExitProg": Value Change {
            n1971 = event-data() -> ()  [unwired: 1 in, 6 out]
            n1972 = call <vilib>:"Add State(s) to Queue__jki_lib_state_machine.vi"("State(s) in Front (\"\")"="Exit" ("State(s) in Front (\"\")"), "State(s) in (\"\")"=w4397) -> ("States Out"=w4396:string)  [unwired: 13 in]
          }
          event Panel Close? {
            n1973 = event-data() -> ()  [unwired: 1 in, 1 out]
            n1974 = event-data("Discard?"=TRUE) -> ()  [unwired: 1 in, 1 out]
            n1975 = call <vilib>:"Add State(s) to Queue__jki_lib_state_machine.vi"("State(s) in Front (\"\")"="Exit", "State(s) in (\"\")"=w4405) -> ("States Out"=w4404:string)  [unwired: 13 in]
          }
        }
      }
      frame "---------- Core ----------" {
        # "Do not put any code in this frame.\n(it is a separator no-op)"
        n1976 = call <vilib>:"Add State(s) to Queue__jki_lib_state_machine.vi"("State(s) in (\"\")"=w4409) -> ("States Out"=w4408:string)  [unwired: 14 in]
      }
      frame Default {
        w4419 = 42 items=["No error", "Argument error", "Memory is full", "Out of zone", "End of file", "File already open", "Generic file I/O error", "File not found", "File permission error", "Disk is full", "Duplicate path", "Too many files open", "System feature not enabled", "Resource file not found", "Cannot add resource", "Resource not found", "Image not found", "Image memory error", "Pen does not exist", "Config type invalid", "Config token not found", "Config parse error", "Config memory error", "Bad external code format", "Bad external code offset", "External code not present", "Null window", "Destroy window error", "Null menu", "Print aborted", "Bad print record", "Print driver error", "Windows error during printing", "Memory error during printing", "Print dialog error", "Generic print error", "Invalid device refnum", "Device not found", "Device parameter error", "Device unit error", "Cannot open device", "Device call aborted", "Generic error", "Cancelled by user", "Object ID too low", "Object ID too high", "Object not in heap", "Unknown heap", "Unknown object (invalid DefProc)", "Unknown object (DefProc not in table)", "Message out of range", "Invalid (null) method", "Unknown message", "Manager call not supported", "Bad address", "Network operation in progress", "Network operation timed out", "Connection is busy", "Network attribute not supported", "Network error", "Address in use", "System out of memory", "Connection aborted", "Connection refused", "Not connected", "Already connected", "Connection closed", "Initialization error (interapplication manager)", "Bad occurrence", "Wait on unbound occurrence handler", "Occurrence queue overflow", "Datalog type conflict", "Unused", "Unrecognized type (interapplication manager)", "Memory corrupt", "Failed to make temporary DLL", "Old CIN version", "Drag socket not found", "Failed to load drop-object", "Failed to register OLE object", "Failed to release OLE object", "Format specifier type mismatch", "Unknown format specifier", "Too few format specifiers", "Too many format specifiers", "Scan failed", "Newer CIN version", "Error converting to variant", "Runtime menu error", "Password tampered", "Variant attribute not found", "Incompatible variant data type", "Event data is not available", "Event Store is not present", "Occurrence is not found", "Event Queue is not created", "Event info is not available", "Refnum passed is NULL", "Error retrieving Class GUID", "Error retrieving CoClass GUID", "Error retrieving TypeLib GUID.", "Bad built application magic bytes.", "Specific driver is different from the specific driver associated with the Logical Name.", "There is no session opened to the class driver.", "Max Error", "MAX - Error with config objects", "MAX - Error loading configuration", "MAX - Group not supported"]
        # "Current State"
        # "Do not delete, rename, or modify this frame.\n(this is used to capture unhandled states and typos)"
        # "Handle mistyped state name (developer tool)"
        n1977 = Format Into String(format string="Software Exception: Unhandled State \"%s\"." ("message"), error in=w4415, w4410) -> (resulting string=w4418:string, error out=w4417:errorcluster)  [unwired: 1 in]
        n1978 = call <vilib>:"Error Cluster From Error Code.vi"("show call chain? (False)"=TRUE, "error in (no error)"=w4417, "error message (\"\")"=w4418, "error code (0)"=w4419) -> ("error out"=w4416:errorcluster)  [unwired: 5 in]
        n1979 = call <vilib>:"Add State(s) to Queue__jki_lib_state_machine.vi"("State(s) in (\"\")"=w4414) -> ("States Out"=w4413:string)  [unwired: 14 in]
      }
      frame "Error Handler" {
        # "Unhandled Error -- Display it"
        # "Handle any errors here.\nYou can also output any states to clean-up after errors occur"
        # "Clear error"
        n1980 = call <vilib>:"General Error Handler.vi"("error in (no error)"=w4422) -> ()  [unwired: 10 in, 5 out]
        n1981 = call <vilib>:"Add State(s) to Queue__jki_lib_state_machine.vi"("State(s) in Front (\"\")"="/* Post Error States", "State(s) in (\"\")"=w4426) -> ("States Out"=w4425:string)  [unwired: 13 in]
      }
      frame "Exit" {
        # "Do not put any code in this frame.\n(No errors that occur here will be handled.)"
        n1982 = call <vilib>:"Add State(s) to Queue__jki_lib_state_machine.vi"("State(s) in (\"\")"=w4431) -> ("States Out"=w4430:string)  [unwired: 14 in]
      }
      frame "---------- Data ----------" {
        # "Do not put any code in this frame.\n(It is a separator no-op. You can make a copy of this frame to create a new Data frame)"
        n1983 = call <vilib>:"Add State(s) to Queue__jki_lib_state_machine.vi"("State(s) in (\"\")"=w4435) -> ("States Out"=w4434:string)  [unwired: 14 in]
      }
      frame "Data: Initialize" {
        w4438 = T25 {"Current VI Reference"=refnum, "Close Panel on Exit?"=FALSE}  # Core
        n1984 = while {
          tunnel: [w4445] -> w4437
          tunnel: [w4443] -> w4436
          stop <- w4446 stop-if-true
          n1985 = Wait Until Next ms Multiple(millisecond multiple=u32 100) -> ()  [unwired: 1 out]
          n1986 = local read "Initialization Complete"() -> (w4446:bool)
          n1987 = local read "Data Out Array"() -> (w4443:T6)
          n1988 = local read "Agilent Refs"() -> (w4445:refnum<visa-resource-name>[])
        }
        n1989 = Bundle("Core"=w4438, "Agilent Refs"=w4437, "Data Out Array"=w4436) -> (w4440:T35)  [unwired: 1 in]
        n1990 = call <vilib>:"Add State(s) to Queue__jki_lib_state_machine.vi"("State(s) in (\"\")"=w4442) -> ("States Out"=w4441:string)  [unwired: 14 in]
      }
      frame "---------- Collect Data ----------" {
        # "Template Separator\n(You can make a copy of, or modify, this frame)"
        n1991 = call <vilib>:"Add State(s) to Queue__jki_lib_state_machine.vi"("State(s) in (\"\")"=w4450) -> ("States Out"=w4449:string)  [unwired: 14 in]
      }
      frame "Read Agilents" {
        # "Try to reduce memory by using notifier"
        n1992 = Unbundle By Name(w4457) -> ("Agilent Refs"=w4459:refnum<visa-resource-name>[], "Data Out Array"=w4458:T6)
        n1993 = local read "Agilent Semaphore"() -> (w4451:T1[])
        n1994 = call "WILT Agilent Read 5 Units.vi"("Agilent Refs"=w4459, "Data Array"=w4458, "Semaphore"=w4451) -> ("Data Out Array"=w4455:T6, "Uncorrected Agilent Data"=→"Uncorrected Agilent Data":dbl[], "Corrected Agilent Data"=→"Corrected Agilent Data":dbl[])  [unwired: 13 in, 1 out]
        "Agilent Data Out" <- w4455
        n1995 = Bundle By Name(cluster=w4457, "Data Out Array"=w4455) -> (w4456:T35)
        n1996 = call <vilib>:"Add State(s) to Queue__jki_lib_state_machine.vi"("State(s) in (\"\")"=w4461) -> ("States Out"=w4460:string)  [unwired: 14 in]
      }
    }
    n1997 = local read "Debug 2"() -> (w4359:bool)
    n1998 = case shown="True" w4359 {
      tunnel: w4362 -> [_ w4377]
      tunnel: [w4372 w4374] -> w4360
      tunnel: w4361 -> [w4372 w4376]
      frame False {
      }
      frame True {
        n1999 = Build Array (concatenate)(w4376, w4377) -> (w4373:string[])
        "Test State array 3" <- w4373
        n2000 = Array Size(array=w4373) -> (size(s)=w4375:i32)
        n2001 = case shown="100" w4375 {
          tunnel: [w4378 w4381] -> w4374
          tunnel: w4373 -> [w4378 w4382]
          frame 0, Default {
          }
          frame 100 {
            n2002 = Delete From Array(array=w4382, length=5, index=0) -> (array with subset deleted=w4381:string[])  [unwired: 1 out]
          }
        }
      }
    }
  }
  n2003 = while "DAQ State Machine" {
    shift-right: [w4474] -> _
    shift-left: _ -> [w4473]
    shift-right: [w4477] -> w42
    shift-left: w41 -> [w4472]
    shift-right: [w4476] -> _
    shift-left: w50 -> [w4478]
    shift-right: [w4469] -> _
    shift-left: string[] [] -> [w4470]
    tunnel: w44 -> [w4464]
    tunnel: [w4463] -> w45
    tunnel: w29 -> [w4462]
    stop <- w4475 stop-if-true
    # "DAQ Save"
    n2004 = call <vilib>:"Parse State Queue__jki_lib_state_machine.vi"("State Queue"=w4478, "Error In (no error)"=w4472) -> ("Remaining States"=w4480:string, "Current State"=w4471:string, "Arguments"=w4479:string)  [unwired: 11 in]
    n2005 = Multiply(x=1000, y="Save Rate (Seconds)") -> (x*y=w4465:i32)
    n2006 = case shown="\"Update Filenames\"" w4471 {
      selector: w4471 -> [_ _ w4522 _ _ _ _ _ _ _]
      tunnel: w4480 -> [w4499 w4520 w4526 w4539 w4545 w4550 w4559 w4572 w4584 w4606]
      tunnel: w4479 -> [_ _ _ _ _ _ _ _ _ _]
      tunnel: w4473 -> [w4497 w4517 w4524 w4536 w4543 w4547 _ w4565 w4581 w4604]
      tunnel: [w4496 w4518 w4528 errorcluster {"status"=FALSE, "code"=0, "source"=""} ("error out") w4542 w4548 w4556 w4567 w4582 w4594] -> w4477
      tunnel: w4472 -> [w4495 w4518 w4527 w4535 w4542 w4548 w4556 w4568 w4582 w4591]
      tunnel: [w4498 w4519 w4525 w4538 w4544 w4549 w4558 w4571 w4583 w4605] -> w4476
      tunnel: [_ _ _ _ TRUE _ _ _ _ _] -> w4475
      tunnel: [w4494 w4517 w4524 w4536 w4543 w4547 w4557 w4565 w4581 w4603] -> w4474
      tunnel: w4465 -> [w4493 _ _ _ _ _ _ _ _ _]
      tunnel: w4464 -> [w4492 w4516 w4521 w4533 w4540 w4546 w4552 w4566 w4580 w4597]
      tunnel: [w4492 w4516 w4521 w4533 w4540 w4546 w4552 w4566 w4580 w4596] -> w4463
      tunnel: w4462 -> [_ _ _ _ _ _ _ _ _ w4592]
      frame "", "Idle" {
        n2007 = event shown="[2] Panel Close?" {
          selector: _ -> [_ _ _]
          dyn-events: _ -> [_ _ _]
          timeout: w4493 -> [_ _ _]
          tunnel: w4499 -> [w4504 w4506 w4515]
          tunnel: [w4503 w4507 w4514] -> w4498
          tunnel: w4497 -> [w4501 w4509 w4512]
          tunnel: [w4502 w4505 w4513] -> w4496
          tunnel: w4495 -> [w4502 w4505 w4513]
          tunnel: [w4501 w4509 w4512] -> w4494
          event Timeout {
            n2008 = event-data() -> ()  [unwired: 1 in, 1 out]
            n2009 = call <vilib>:"Add State(s) to Queue__jki_lib_state_machine.vi"("State(s) in Front (\"\")"="Update Filenames" ("State(s) in Front (\"\")"), "State(s) in (\"\")"=w4504) -> ("States Out"=w4503:string)  [unwired: 13 in]
          }
          event "ExitProg": Value Change {
            n2010 = event-data() -> ()  [unwired: 1 in, 6 out]
            n2011 = call <vilib>:"Add State(s) to Queue__jki_lib_state_machine.vi"("State(s) in Front (\"\")"="Exit" ("State(s) in Front (\"\")"), "State(s) in (\"\")"=w4506) -> ("States Out"=w4507:string)  [unwired: 13 in]
          }
          event Panel Close? {
            n2012 = event-data() -> ()  [unwired: 1 in, 1 out]
            n2013 = event-data("Discard?"=TRUE) -> ()  [unwired: 1 in, 1 out]
            n2014 = call <vilib>:"Add State(s) to Queue__jki_lib_state_machine.vi"("State(s) in Front (\"\")"="Exit", "State(s) in (\"\")"=w4515) -> ("States Out"=w4514:string)  [unwired: 13 in]
          }
        }
      }
      frame "---------- Core ----------" {
        # "Do not put any code in this frame.\n(it is a separator no-op)"
        n2015 = call <vilib>:"Add State(s) to Queue__jki_lib_state_machine.vi"("State(s) in (\"\")"=w4520) -> ("States Out"=w4519:string)  [unwired: 14 in]
      }
      frame Default {
        w4531 = 42 items=["No error", "Argument error", "Memory is full", "Out of zone", "End of file", "File already open", "Generic file I/O error", "File not found", "File permission error", "Disk is full", "Duplicate path", "Too many files open", "System feature not enabled", "Resource file not found", "Cannot add resource", "Resource not found", "Image not found", "Image memory error", "Pen does not exist", "Config type invalid", "Config token not found", "Config parse error", "Config memory error", "Bad external code format", "Bad external code offset", "External code not present", "Null window", "Destroy window error", "Null menu", "Print aborted", "Bad print record", "Print driver error", "Windows error during printing", "Memory error during printing", "Print dialog error", "Generic print error", "Invalid device refnum", "Device not found", "Device parameter error", "Device unit error", "Cannot open device", "Device call aborted", "Generic error", "Cancelled by user", "Object ID too low", "Object ID too high", "Object not in heap", "Unknown heap", "Unknown object (invalid DefProc)", "Unknown object (DefProc not in table)", "Message out of range", "Invalid (null) method", "Unknown message", "Manager call not supported", "Bad address", "Network operation in progress", "Network operation timed out", "Connection is busy", "Network attribute not supported", "Network error", "Address in use", "System out of memory", "Connection aborted", "Connection refused", "Not connected", "Already connected", "Connection closed", "Initialization error (interapplication manager)", "Bad occurrence", "Wait on unbound occurrence handler", "Occurrence queue overflow", "Datalog type conflict", "Unused", "Unrecognized type (interapplication manager)", "Memory corrupt", "Failed to make temporary DLL", "Old CIN version", "Drag socket not found", "Failed to load drop-object", "Failed to register OLE object", "Failed to release OLE object", "Format specifier type mismatch", "Unknown format specifier", "Too few format specifiers", "Too many format specifiers", "Scan failed", "Newer CIN version", "Error converting to variant", "Runtime menu error", "Password tampered", "Variant attribute not found", "Incompatible variant data type", "Event data is not available", "Event Store is not present", "Occurrence is not found", "Event Queue is not created", "Event info is not available", "Refnum passed is NULL", "Error retrieving Class GUID", "Error retrieving CoClass GUID", "Error retrieving TypeLib GUID.", "Bad built application magic bytes.", "Specific driver is different from the specific driver associated with the Logical Name.", "There is no session opened to the class driver.", "Max Error", "MAX - Error with config objects", "MAX - Error loading configuration", "MAX - Group not supported"]
        # "Current State"
        # "Do not delete, rename, or modify this frame.\n(this is used to capture unhandled states and typos)"
        # "Handle mistyped state name (developer tool)"
        n2016 = Format Into String(format string="Software Exception: Unhandled State \"%s\"." ("message"), error in=w4527, w4522) -> (resulting string=w4530:string, error out=w4529:errorcluster)  [unwired: 1 in]
        n2017 = call <vilib>:"Error Cluster From Error Code.vi"("show call chain? (False)"=TRUE, "error in (no error)"=w4529, "error message (\"\")"=w4530, "error code (0)"=w4531) -> ("error out"=w4528:errorcluster)  [unwired: 5 in]
        n2018 = call <vilib>:"Add State(s) to Queue__jki_lib_state_machine.vi"("State(s) in (\"\")"=w4526) -> ("States Out"=w4525:string)  [unwired: 14 in]
      }
      frame "Error Handler" {
        # "Unhandled Error -- Display it"
        # "Handle any errors here.\nYou can also output any states to clean-up after errors occur"
        # "Clear error"
        n2019 = call <vilib>:"General Error Handler.vi"("error in (no error)"=w4535) -> ()  [unwired: 10 in, 5 out]
        n2020 = call <vilib>:"Add State(s) to Queue__jki_lib_state_machine.vi"("State(s) in Front (\"\")"="/* Post Error States", "State(s) in (\"\")"=w4539) -> ("States Out"=w4538:string)  [unwired: 13 in]
      }
      frame "Exit" {
        # "Do not put any code in this frame.\n(No errors that occur here will be handled.)"
        n2021 = call <vilib>:"Add State(s) to Queue__jki_lib_state_machine.vi"("State(s) in (\"\")"=w4545) -> ("States Out"=w4544:string)  [unwired: 14 in]
      }
      frame "---------- Data ----------" {
        # "Do not put any code in this frame.\n(It is a separator no-op. You can make a copy of this frame to create a new Data frame)"
        n2022 = call <vilib>:"Add State(s) to Queue__jki_lib_state_machine.vi"("State(s) in (\"\")"=w4550) -> ("States Out"=w4549:string)  [unwired: 14 in]
      }
      frame "Data: Initialize" {
        w4555 = T25 {"Current VI Reference"=refnum, "Close Panel on Exit?"=FALSE}  # Core
        n2023 = while {
          tunnel: [w4563] -> w4554
          tunnel: [w4562] -> w4553
          tunnel: [w4560] -> w4551
          stop <- w4564 stop-if-true
          w4563 = bool[] [TRUE, TRUE, TRUE, TRUE, TRUE, TRUE, TRUE, TRUE, TRUE, TRUE, TRUE, TRUE, TRUE, TRUE, TRUE, TRUE, TRUE, TRUE, TRUE, TRUE, TRUE, TRUE, TRUE, TRUE, TRUE, TRUE, TRUE, TRUE, TRUE, TRUE, TRUE, TRUE, TRUE, TRUE, TRUE, TRUE, TRUE, TRUE, TRUE, TRUE, TRUE, TRUE, TRUE, TRUE, TRUE, TRUE, TRUE, TRUE, TRUE, TRUE, TRUE, TRUE, TRUE, TRUE, TRUE, TRUE]  # First Time Through?
          n2024 = Wait Until Next ms Multiple(millisecond multiple=u32 100) -> ()  [unwired: 1 out]
          n2025 = local read "Initialization Complete"() -> (w4564:bool)
          n2026 = local read "File Refnums"() -> (w4560:refnum<file>[])
          n2027 = local read "File Locations"() -> (w4562:T17[])
        }
        n2028 = Bundle("Core"=w4555, "First Time Through?"=w4554, "File Locations"=w4553, "File Refnums"=w4551) -> (w4557:T36)  [unwired: 1 in]
        n2029 = call <vilib>:"Add State(s) to Queue__jki_lib_state_machine.vi"("State(s) in (\"\")"=w4559) -> ("States Out"=w4558:string)  [unwired: 14 in]
      }
      frame "Prepare for Save" {
        n2030 = flat-sequence {
          tunnel: w4568 -> [w4573]
          tunnel: [w4575] -> w4570
          tunnel: [w4577] -> w4569
          tunnel: w4565 -> [w4576]
          tunnel: [w4578] -> w4567
          tunnel: w4570 -> [w4578]
          tunnel: w4569 -> [w4579]
          frame #0 {
            # "Wait for the save loop to \ncomplete, then update\nthe new save locations"
            n2031 = Unbundle By Name(w4576) -> ("File Locations"=w4577:T17[])
            n2032 = call "UTILITY Delay mS.vi"("Error In"=w4573, "milliseconds to wait"=u32 5000) -> ("Error Out"=w4575:errorcluster)  [unwired: 13 in]
          }
          frame #1 {
            n2033 = local write "File Locations"(w4579) -> ()
          }
        }
        n2034 = call <vilib>:"Add State(s) to Queue__jki_lib_state_machine.vi"("State(s) in (\"\")"=w4572) -> ("States Out"=w4571:string)  [unwired: 14 in]
      }
      frame "---------- Collect Data ----------" {
        # "Template Separator\n(You can make a copy of, or modify, this frame)"
